vi "Edit Module Timeout.vi"(7 "Theme":bool, 8 "error in":errorcluster, 11 "Value":variant) -> (0 "error out":errorcluster, 2 "Canceled":bool, 3 "New Module Timeout":i32)   [LabVIEW 2019, in "Panther Dashboard.lvlib"]
uses:
  Panther Dashboard.lvlib
panel:
  in  "Reset":bool
  in  "Continue":bool
  in  "Cancel":bool
  in  "Module Timeout":i32
  # "- The 'Module Timeout--constant.vi' in the DQMH Framework serves as a mechanism to control the maximum time that all the 'Request and Wait for Reply' waits for a response.\n- By default, this timeout value is set to 5000 milliseconds (ms), which translates to 5 seconds.\n\n**When to Use Custom Timeout for a DQMH module:**\n\n- Consider altering the Timeout value for a DQMH Module in the following scenarios:\n    - If a module is inherently slow-responding due to complex calculations or external interactions, you might need to increase the Module Timeout to prevent premature timeouts.\n    - Conversely, if you're confident that a module's response should typically be much faster than 5 seconds, you could decrease the Timeout to optimize performance and avoid unnecessary waiting.\n\nNOTES:\n\n- Exercise caution when reducing the timeout excessively, as it could lead to premature timeouts and disrupt your application's functionality."
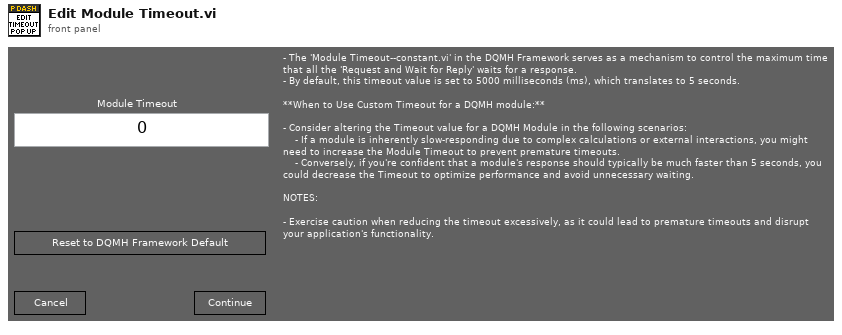
[diagram p1: front panel]
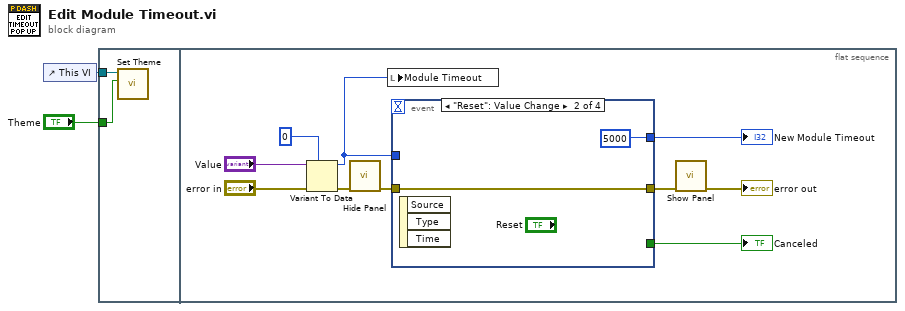
[diagram p0: block diagram]
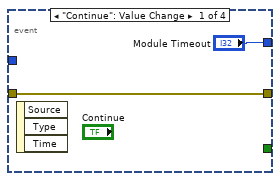
[diagram p2: hidden frame]
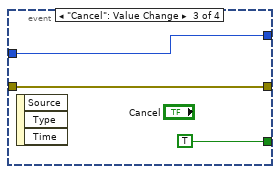
[diagram p3: hidden frame]
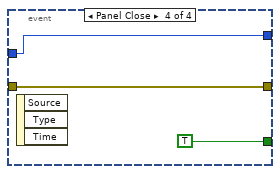
[diagram p4: hidden frame]
diagram:
  n1 = control-ref of="This VI"() -> (w2:refnum<vi>)
  n2 = flat-sequence {
    tunnel: w2 -> [w4]
    tunnel: "Theme" -> [w3]
    frame #0 {
      n3 = call "Set Theme.vi"("Dark?"=w3, "VI in"=w4) -> ()  [unwired: 10 in]
    }
    frame #1 {
      n4 = Variant To Data(error in="error in", type=0, Variant="Value") -> (data=w9:i32, error out=w12:errorcluster)
      n5 = call "Hide Panel.vi"("error in (no error)"=w12) -> ("error out"=w13:errorcluster)  [unwired: 10 in]
      n6 = local write "Module Timeout"(w9) -> ()
      n7 = event shown="[1] \"Reset\": Value Change" {
        selector: _ -> [_ _ _ _]
        dyn-events: _ -> [_ _ _ _]
        timeout: _ -> [_ _ _ _]
        tunnel: ["Module Timeout" 5000 ("Module Timeout 2") w20 w22] -> w8
        tunnel: w9 -> [_ _ w20 w22]
        tunnel: [w16 w18 w21 w24] -> w14
        tunnel: w13 -> [w16 w18 w21 w24]
        tunnel: [_ _ TRUE ("Cancel Button") TRUE ("Cancel Button")] -> w5
        event "Continue": Value Change {
          n8 = event-data() -> ()  [unwired: 1 in, 3 out]
        }
        event "Reset": Value Change {
          n9 = event-data() -> ()  [unwired: 1 in, 3 out]
        }
        event "Cancel": Value Change {
          n10 = event-data() -> ()  [unwired: 1 in, 3 out]
        }
        event Panel Close {
          n11 = event-data() -> ()  [unwired: 1 in, 3 out]
        }
      }
      "New Module Timeout" <- w8
      "Canceled" <- w5
      n12 = call "Show Panel.vi"("error in (no error)"=w14) -> ("error out"=→"error out":errorcluster)  [unwired: 10 in]
    }
  }
